vi "Get Phys Chan Property.vi"   [LabVIEW 2020, in "SLSC.lvlib"]
doc: "Gets the value of the specified physical channel property from one or more physical channels. You can use an array instance of this VI to get a scalar property from multiple devices with a single call to the VI."
uses:
  <vilib>/SLSC/SLSC.lvlib
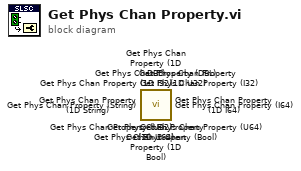
[diagram p0: block diagram]
diagram:
  n1 = call <vilib>:"Get Phys Chan Property (1D U64).vi"() -> ()  [unwired: 13 in, 3 out]
  n2 = call <vilib>:"Get Phys Chan Property (1D U32).vi"() -> ()  [unwired: 13 in, 3 out]
  n3 = call <vilib>:"Get Phys Chan Property (1D String).vi"() -> ()  [unwired: 13 in, 3 out]
  n4 = call <vilib>:"Get Phys Chan Property (1D I64).vi"() -> ()  [unwired: 13 in, 3 out]
  n5 = call <vilib>:"Get Phys Chan Property (1D I32).vi"() -> ()  [unwired: 13 in, 3 out]
  n6 = call <vilib>:"Get Phys Chan Property (1D DBL).vi"() -> ()  [unwired: 13 in, 3 out]
  n7 = call <vilib>:"Get Phys Chan Property (1D Bool).vi"() -> ()  [unwired: 13 in, 3 out]
  n8 = call <vilib>:"Get Phys Chan Property (U64).vi"() -> ()  [unwired: 13 in, 3 out]
  n9 = call <vilib>:"Get Phys Chan Property (U32).vi"() -> ()  [unwired: 13 in, 3 out]
  n10 = call <vilib>:"Get Phys Chan Property (String).vi"() -> ()  [unwired: 13 in, 3 out]
  n11 = call <vilib>:"Get Phys Chan Property (I64).vi"() -> ()  [unwired: 13 in, 3 out]
  n12 = call <vilib>:"Get Phys Chan Property (I32).vi"() -> ()  [unwired: 13 in, 3 out]
  n13 = call <vilib>:"Get Phys Chan Property (DBL).vi"() -> ()  [unwired: 13 in, 3 out]
  n14 = call <vilib>:"Get Phys Chan Property (Bool).vi"() -> ()  [unwired: 13 in, 3 out]
